vi "Stream Chunk.vi"(8 "error in (no error)":errorcluster, 9 "Stream in":refnum<k5>, 10 "Content Chunk":string, 11 "Response in":refnum<class "Response.lvclass">) -> (0 "error out":errorcluster, 1 "Stream out":refnum<k5>, 3 "Response out":refnum<class "Response.lvclass">)   [LabVIEW 2020, in "HTTP Utils.lvlib" / "Response.lvclass"]
doc: "Allows starting to transfer data when the full buffer is not available at once, possibly due to time or memory constraints. Data can be sent chunks at a time and will be completed by writing an empty string.\n\nDepending on the timeout settings of the remote system, waiting too long between sending chunks may cause the remote system to close the connection with a timeout before the response is completed.\n\nThis method should not be used for holding a connection open to continually send data long-term."
uses:
  Response.lvclass
  Response.lvclass/Response.ctl
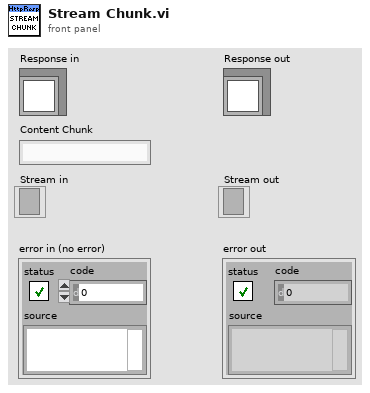
[diagram p1: front panel]
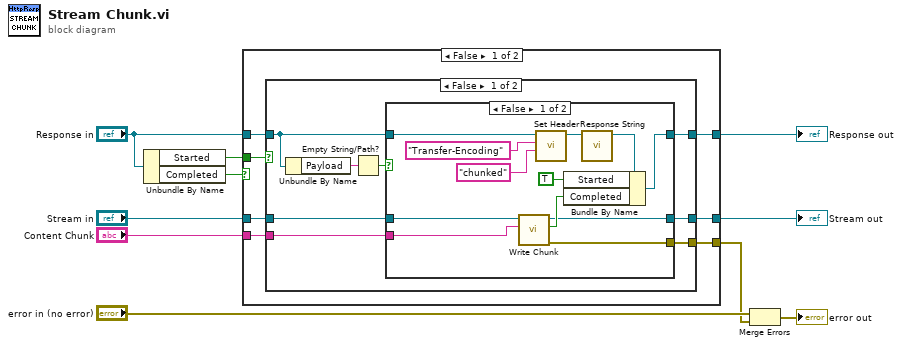
[diagram p0: block diagram]
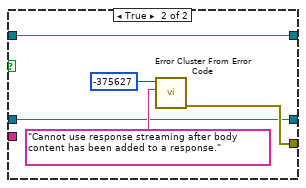
[diagram p2: hidden frame]
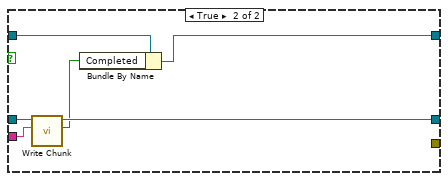
[diagram p3: hidden frame]
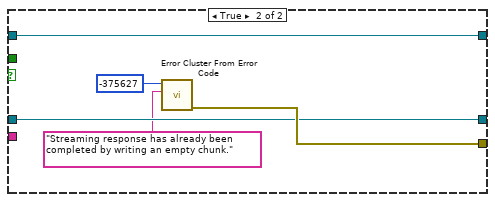
[diagram p4: hidden frame]
diagram:
  n1 = Unbundle By Name("Response in") -> ("Started"=w10:bool, "Completed"=w1:bool)
  n2 = case shown="False" w1 {
    tunnel: w10 -> [w17 _]
    tunnel: "Response in" -> [w16 w52]
    tunnel: [w15 w52] -> w8
    tunnel: "Stream in" -> [w14 w51]
    tunnel: "Content Chunk" -> [w13 _]
    tunnel: [w12 w51] -> w5
    tunnel: [w11 w53] -> w3
    frame False {
      n3 = case shown="False" w17 {
        tunnel: w16 -> [w22 w48]
        tunnel: [w21 w44] -> w15
        tunnel: [w24 _] -> w11
        tunnel: w14 -> [w23 w47]
        tunnel: w13 -> [w20 w45]
        tunnel: [w19 w46] -> w12
        frame False {
          n4 = Unbundle By Name(w22) -> ("Payload"=w25:string)
          n5 = Empty String/Path?(string/path=w25) -> (empty?=w18:bool)
          n6 = case shown="False" w18 {
            tunnel: [w26 w40] -> w24
            tunnel: w23 -> [w30 w38]
            tunnel: w22 -> [w37 w39]
            tunnel: [w32 w39] -> w21
            tunnel: w20 -> [w28 _]
            tunnel: [w27 w38] -> w19
            frame False {
              n7 = call "Write Chunk.vi"("Content Chunk"=w28, "Stream in"=w30) -> ("error out"=w26:errorcluster, "Done"=w29:bool, "Stream out"=w27:refnum<k5>)  [unwired: 7 in]
              n8 = call "Set Header.vi"("Value"="chunked" ("Header"), "Header"="Transfer-Encoding", "Response in"=w37) -> ("Response out"=w36:refnum<class "Response.lvclass">)  [unwired: 6 in, 2 out]
              n9 = call-dynamic "Response String.vi"("Response in"=w36) -> ("Response out"=w33:refnum<class "Response.lvclass">)  [unwired: 8 in, 2 out]
              n10 = Bundle By Name(cluster=w33, "Started"=TRUE ("Streaming.Started"), "Completed"=w29) -> (w32:refnum<class "Response.lvclass">)
            }
            frame True {
              n11 = call <vilib>:"Error Cluster From Error Code.vi"("error message (\"\")"="Cannot use response streaming after body content has been added to a response." ("error message (\"\")"), "error code (0)"=-375627) -> ("error out"=w40:errorcluster)  [unwired: 7 in]
            }
          }
        }
        frame True {
          n12 = call "Write Chunk.vi"("Content Chunk"=w45, "Stream in"=w47) -> ("Done"=w43:bool, "Stream out"=w46:refnum<k5>)  [unwired: 7 in, 1 out]
          n13 = Bundle By Name(cluster=w48, "Completed"=w43) -> (w44:refnum<class "Response.lvclass">)
        }
      }
    }
    frame True {
      n14 = call <vilib>:"Error Cluster From Error Code.vi"("error message (\"\")"="Streaming response has already been completed by writing an empty chunk." ("error message (\"\")"), "error code (0)"=-375627) -> ("error out"=w53:errorcluster)  [unwired: 7 in]
    }
  }
  "Response out" <- w8
  "Stream out" <- w5
  n15 = Merge Errors("error in (no error)", w3) -> (→"error out":errorcluster)
